vi "make_electrode_array (SubVI).vi"(11 "Electrode settings:":T1={"DC volts (V):\n"=[], "Electrode to sweep:"=0, "start volt (V)"=0.0, "stop volt (V) "=0.0, "# V Steps"=1, "start freq (Hz)"=41.0, "stop freq (Hz) "=41.0, "# F steps"=1, "start DC (V)"=0.0, "stop DC (V)"=0.0, "# DC steps "=1, "Digitize electrode\ndrives?"=FALSE, "Sweep electrode?"=FALSE, "Add 0.5*V DC \noffset for amp?"=FALSE}) -> (3 "Tot Electrode Arr":dbl[][](array[numeric]))   [LabVIEW 2014]
panel:
  # "0"
  # "1"
  # "2"
  # "3"
  # "4"
  # "5"
  # "6"
  # "7"
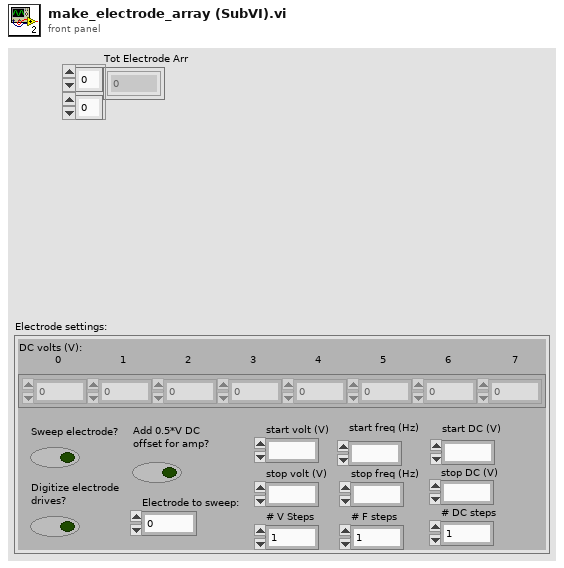
[diagram p1: front panel]
types:
  T1 = cluster{"DC volts (V):\n":dbl[], "Electrode to sweep:":i32, "start volt (V)":ext, "stop volt (V) ":ext, "# V Steps":i32, "start freq (Hz)":ext, "stop freq (Hz) ":ext, "# F steps":i32, "start DC (V)":ext, "stop DC (V)":ext, "# DC steps ":i32, "Digitize electrode\ndrives?":bool, "Sweep electrode?":bool, "Add 0.5*V DC \noffset for amp?":bool}
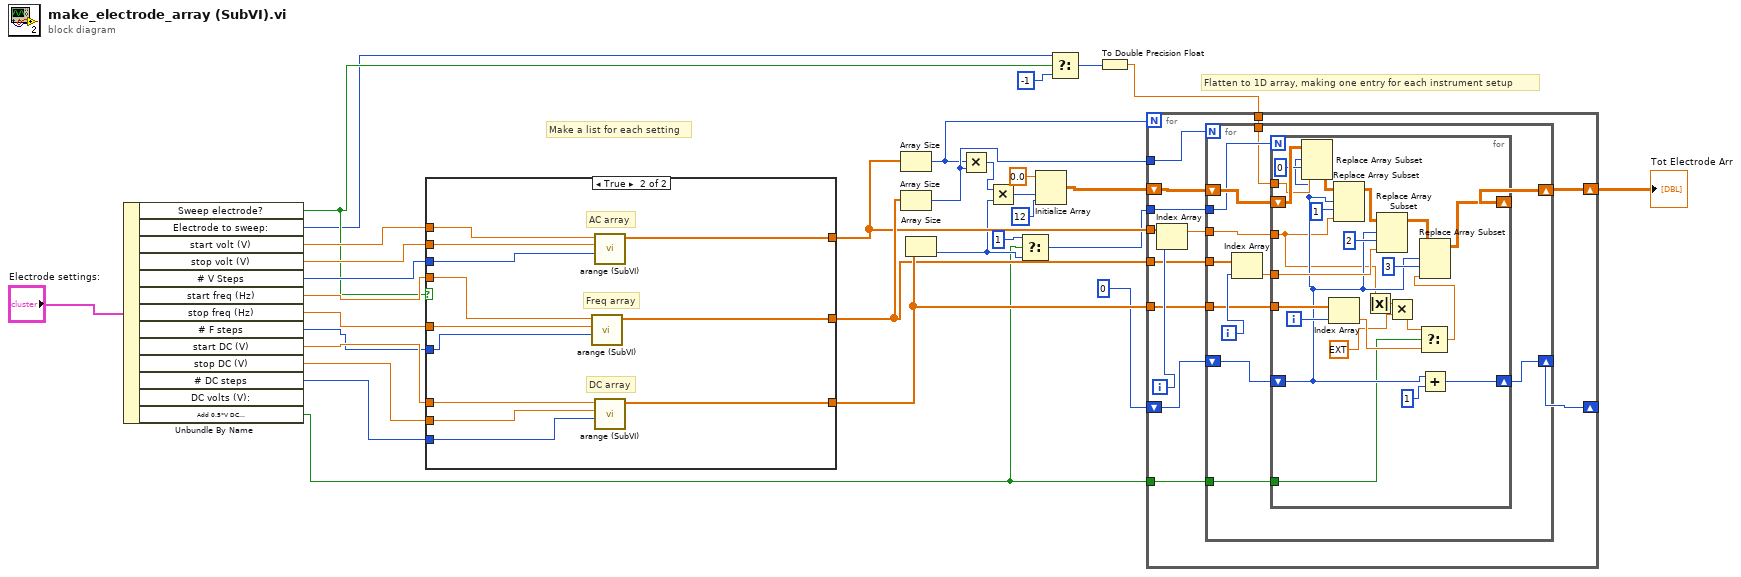
[diagram p0: block diagram]
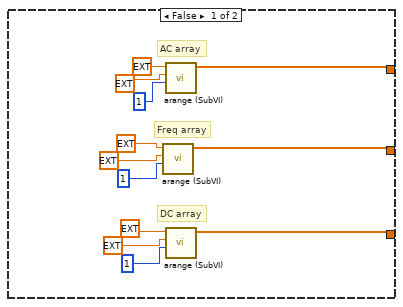
[diagram p2: hidden frame]
diagram:
  # "Make a list for each setting"
  # "Flatten to 1D array, making one entry for each instrument setup"
  n1 = Unbundle By Name("Electrode settings:") -> ("Sweep electrode?"=w10:bool, "Electrode to sweep:"=w9:i32, "start volt (V)"=w23:ext, "stop volt (V)"=w24:ext, "# V Steps"=w25:i32, "start freq (Hz)"=w26:ext, "stop freq (Hz)"=w27:ext, "# F steps"=w28:i32, "start DC (V)"=w29:ext, "stop DC (V)"=w30:ext, "# DC steps"=w31:i32, "Add 0.5*V DC \noffset for amp?"=w1:bool)  [unwired: 1 out]
  n2 = case shown="True" w10 {
    tunnel: w23 -> [_ w55]
    tunnel: w24 -> [_ w54]
    tunnel: w25 -> [_ w53]
    tunnel: w26 -> [_ w52]
    tunnel: w27 -> [_ w51]
    tunnel: w28 -> [_ w50]
    tunnel: w29 -> [_ w49]
    tunnel: w30 -> [_ w48]
    tunnel: w31 -> [_ w47]
    tunnel: [w34 w46] -> w18
    tunnel: [w33 w45] -> w19
    tunnel: [w32 w44] -> w20
    frame False {
      # "DC array"
      # "Freq array"
      # "AC array"
      n3 = call "arange (SubVI).vi"("# Steps"=1, "stop"=ext 0.0, "start"=ext 0.0) -> ("Array"=w33:ext[])  [unwired: 8 in]
      n4 = call "arange (SubVI).vi"("# Steps"=1, "stop"=ext 0.0, "start"=ext 0.0) -> ("Array"=w34:ext[])  [unwired: 8 in]
      n5 = call "arange (SubVI).vi"("# Steps"=1, "stop"=ext 0.0, "start"=ext 0.0) -> ("Array"=w32:ext[])  [unwired: 8 in]
    }
    frame True {
      # "DC array"
      # "Freq array"
      # "AC array"
      n6 = call "arange (SubVI).vi"("# Steps"=w50, "stop"=w51, "start"=w52) -> ("Array"=w45:ext[])  [unwired: 8 in]
      n7 = call "arange (SubVI).vi"("# Steps"=w53, "stop"=w54, "start"=w55) -> ("Array"=w46:ext[])  [unwired: 8 in]
      n8 = call "arange (SubVI).vi"("# Steps"=w47, "stop"=w48, "start"=w49) -> ("Array"=w44:ext[])  [unwired: 8 in]
    }
  }
  n9 = Array Size(array=w18) -> (size(s)=w21:i32)
  n10 = Array Size(array=w19) -> (size(s)=w22:i32)
  n11 = Array Size(array=w20) -> (size(s)=w4:i32)
  n12 = Multiply(x=w21, y=w22) -> (x*y=w12:i32)
  n13 = Multiply(x=w12, y=w4) -> (x*y=w13:i32)
  n14 = Select(t=1, s=w1, f=w4) -> (s? t:f=w3:i32)
  n15 = Initialize Array(0.0 ("element"), w13, 12 ("dimension size")) -> (w15:dbl[][])
  n16 = Select(t=w9, s=w10, f=-1) -> (s? t:f=w7:i32)
  n17 = To Double Precision Float(number=w7) -> (double precision float=w6:dbl)
  n18 = for {
    N: w21 -> [_]
    shift-right: [w58] -> _
    shift-left: 0 ("disabled index (row)") -> [w59]
    shift-right: [w67] -> w17
    shift-left: w15 -> [w68]
    tunnel: w18 -> [w66]
    tunnel: w19 -> [w63]
    tunnel: w20 -> [w62]
    tunnel: w22 -> [w61]
    tunnel: w3 -> [w60]
    tunnel: w6 -> [w57]
    tunnel: w1 -> [w56]
    i -> [w64]
    n19 = Index Array(array=w66, index=w64) -> (element=w65:ext)
    n20 = for {
      N: w61 -> [_]
      tunnel: w65 -> [w78]
      tunnel: w63 -> [w77]
      tunnel: w62 -> [w74]
      tunnel: w60 -> [w73]
      shift-right: [w79] -> w67
      shift-left: w68 -> [w80]
      shift-right: [w71] -> w58
      shift-left: w59 -> [w72]
      tunnel: w57 -> [w70]
      tunnel: w56 -> [w69]
      i -> [w76]
      n21 = Index Array(array=w77, index=w76) -> (element=w75:ext)
      n22 = for {
        N: w73 -> [_]
        tunnel: w78 -> [w82]
        tunnel: w75 -> [w98]
        tunnel: w74 -> [w96]
        shift-right: [w88] -> w79
        shift-left: w80 -> [w92]
        shift-right: [w94] -> w71
        shift-left: w72 -> [w89]
        tunnel: w70 -> [w90]
        tunnel: w69 -> [w85]
        i -> [w97]
        n23 = Replace Array Subset(array=w92, new element=w90, index (row)=w89, index (col)=0 ("disabled index (col)")) -> (w93:dbl[][])
        n24 = Index Array(array=w96, index=w97) -> (element=w87:ext)
        n25 = Replace Array Subset(array=w93, new element=w82, index (row)=w89, index (col)=1 ("disabled index (col)")) -> (w102:dbl[][])
        n26 = Absolute Value(x=w82) -> (abs(x)=w81:ext)
        n27 = Replace Array Subset(array=w102, new element=w98, index (row)=w89, index (col)=2 ("disabled index (col)")) -> (w101:dbl[][])
        n28 = Multiply(x=w81, y=ext 1.0) -> (x*y=w84:ext)
        n29 = Select(t=w84, s=w85, f=w87) -> (s? t:f=w86:ext)
        n30 = Replace Array Subset(array=w101, new element=w86, index (row)=w89, index (col)=3 ("disabled index (col)")) -> (w88:dbl[][])
        n31 = Add(x=w89, y=1) -> (x+y=w94:i32)
      }
    }
  }
  "Tot Electrode Arr" <- w17
